vi "test_ReplaceClusterData.vi"() -> ()   [LabVIEW 2013]
uses:
  <vilib>/Utility/sysdir.llb/System Directory Type.ctl
panel:
  out "ArrayOfStrings":string[](array[string])
  out "Value":variant
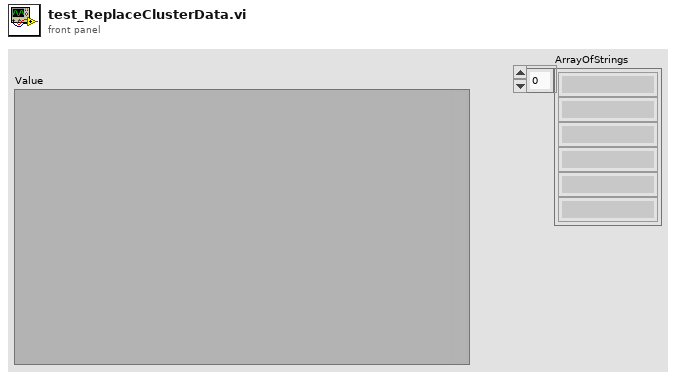
[diagram p1: front panel]
types:
  T1 = typedef "System Directory Type.ctl" = i32
  T2 = cluster{"Numeric":i8, "HomeDir":string, "AppDir":string, "BooleanData":i8, "Process":cluster{"timeout":i32, "run":bool}, "ArrayOfStrings":string[]}
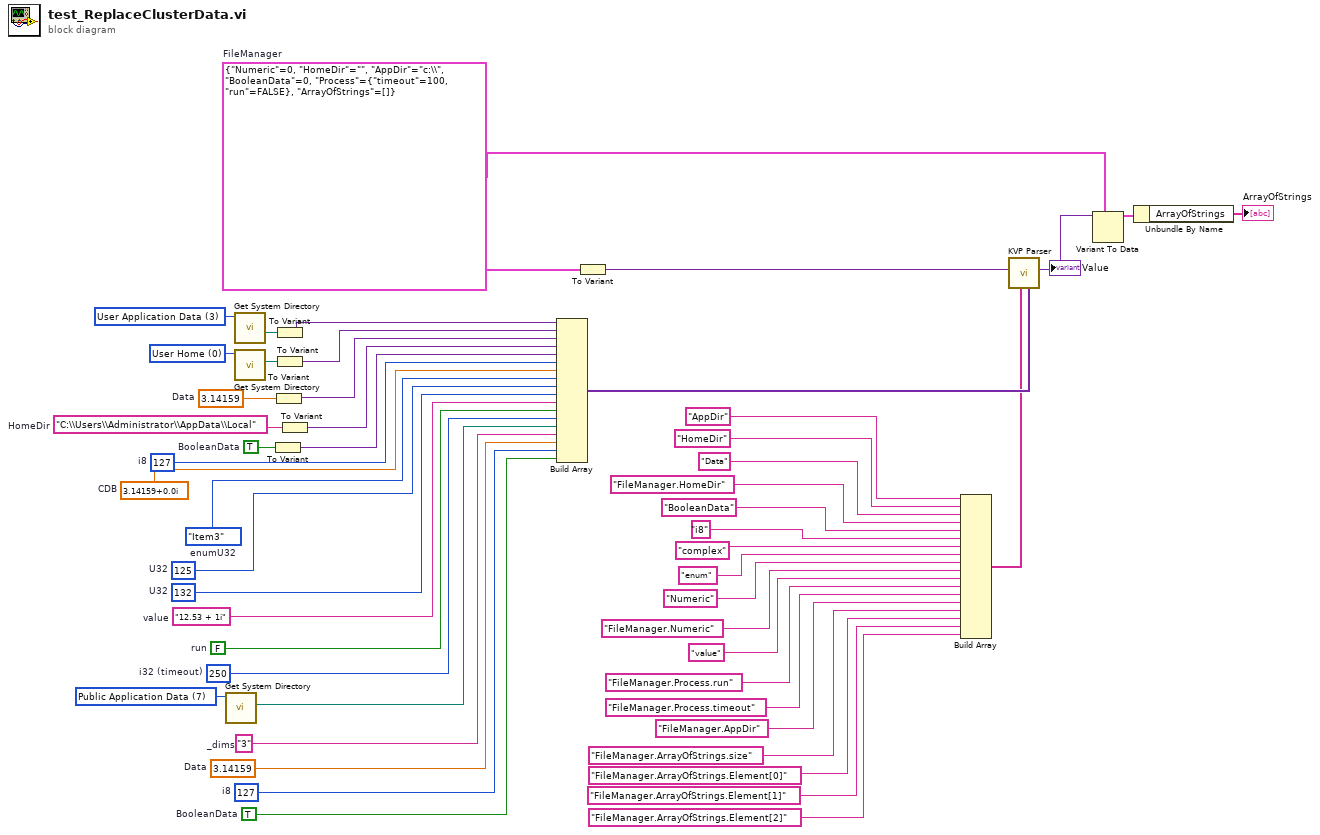
[diagram p0: block diagram]
diagram:
  w8 = TRUE  # BooleanData
  w9 = i8 127  # i8
  w10 = 3.14159  # Data
  w11 = "3"  # _dims
  w17 = T1 7 items=["User Home"=0, "User Desktop"=1, "User Documents"=2, "User Application Data"=3, "User Preferences"=4, "User Temporary"=5, "Public Documents"=6, "Public Application Data"=7, "Public Preferences"=8, "Public Cache"=13, "System Core Libraries"=9, "System Installed Libraries"=10, "Application Files"=11, "Boot Volume Root"=12] ("system directory type")
  w21 = 250  # i32 (timeout)
  w22 = FALSE  # run
  w25 = "12.53 + 1i"  # value
  w26 = u32 132  # U32
  w29 = u32 125  # U32
  w31 = enum32{"Item1", "Item2", "Item3"}."Item3"  # enumU32
  w33 = cdb 3.14159+0.0i  # CDB
  w34 = i8 127  # i8
  w37 = TRUE  # BooleanData
  w41 = "C:\\Users\\Administrator\\AppData\\Local"  # HomeDir
  w42 = 3.14159  # Data
  w49 = T1 0 items=["User Home"=0, "User Desktop"=1, "User Documents"=2, "User Application Data"=3, "User Preferences"=4, "User Temporary"=5, "Public Documents"=6, "Public Application Data"=7, "Public Preferences"=8, "Public Cache"=13, "System Core Libraries"=9, "System Installed Libraries"=10, "Application Files"=11, "Boot Volume Root"=12] ("system directory type")
  w51 = T1 3 items=["User Home"=0, "User Desktop"=1, "User Documents"=2, "User Application Data"=3, "User Preferences"=4, "User Temporary"=5, "Public Documents"=6, "Public Application Data"=7, "Public Preferences"=8, "Public Cache"=13, "System Core Libraries"=9, "System Installed Libraries"=10, "Application Files"=11, "Boot Volume Root"=12] ("system directory type")
  w3 = T2 {"Numeric"=0, "HomeDir"="", "AppDir"="c:\\", "BooleanData"=0, "Process"={"timeout"=100, "run"=FALSE}, "ArrayOfStrings"=[]}  # FileManager
  n1 = call <vilib>:"Get System Directory.vi"("system directory type"=w17) -> ("system directory"=w16:path)  [unwired: 10 in]
  n2 = call <vilib>:"Get System Directory.vi"("system directory type"=w51) -> ("system directory"=w50:path)  [unwired: 10 in]
  n3 = call <vilib>:"Get System Directory.vi"("system directory type"=w49) -> ("system directory"=w48:path)  [unwired: 10 in]
  n4 = To Variant(anything=w37) -> (Variant=w36:variant)
  n5 = To Variant(anything=w42) -> (Variant=w46:variant)
  n6 = To Variant(anything=w50) -> (Variant=w23:variant)
  n7 = To Variant(anything=w48) -> (Variant=w47:variant)
  n8 = To Variant(anything=w41) -> (Variant=w40:variant)
  n9 = Build Array(w23, w47, w46, w40, w36, w34, w33, w31, w29, w26, w25, w22, w21, w16, w11, w10, w9, w8) -> (w14:variant[])
  n10 = To Variant(anything=w3) -> (Variant=w15:variant)
  n11 = Build Array("AppDir", "HomeDir", "Data", "FileManager.HomeDir", "BooleanData", "i8", "complex", "enum", "Numeric", "FileManager.Numeric", "value", "FileManager.Process.run", "FileManager.Process.timeout", "FileManager.AppDir", "FileManager.ArrayOfStrings.size", "FileManager.ArrayOfStrings.Element[0]", "FileManager.ArrayOfStrings.Element[1]", "FileManager.ArrayOfStrings.Element[2]") -> (w13:string[])
  n12 = call "KVP Parser.vi"("Values"=w14, "Keys"=w13, "Default Value"=w15) -> ("Value"=w4:variant)  [unwired: 5 in, 3 out]
  "Value" <- w4
  n13 = Variant To Data(type=w3, Variant=w4) -> (data=w2:T2)  [unwired: 1 in, 1 out]
  n14 = Unbundle By Name(w2) -> ("ArrayOfStrings"=→"ArrayOfStrings":string[])
